vi "Connection Loop.vi"(8 "Timeout":i32=1000, 11 "connection ID":refnum<k5>) -> ()   [LabVIEW 2017]
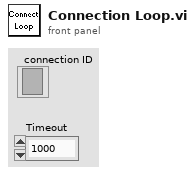
[diagram p1: front panel]
types:
  T1 = enum16{"Add Cnx", "Remove Cnx", "Retrieve List", "Cnx Inited"}
  T2 = cluster{"vi reference":refnum<vi>, "connection ID":refnum<k5>, cluster{"RPC field ID":u16, "Unique ID":u16}}
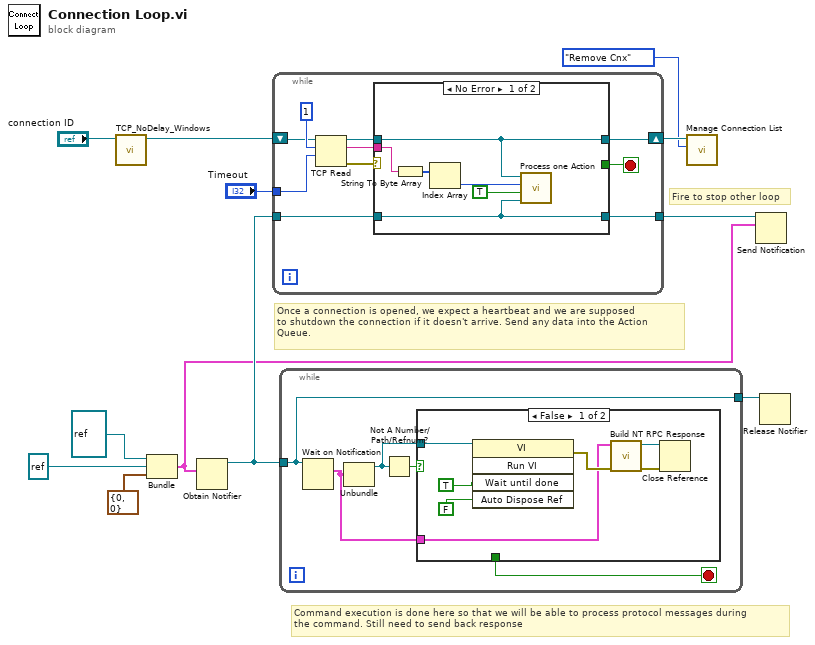
[diagram p0: block diagram]
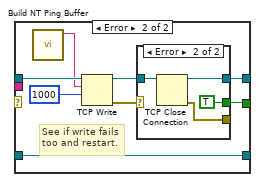
[diagram p3: hidden frame]
diagram:
  # "Command execution is done here so that we will be able to process protocol messages during\nthe command. Still need to send back response"
  # "Fire to stop other loop"
  # "Once a connection is opened, we expect a heartbeat and we are supposed\nto shutdown the connection if it doesn't arrive. Send any data into the Action\nQueue."
  n1 = call <vilib>:"TCP_NoDelay_Windows.vi"("connID"="connection ID") -> ("connID 2"=w1:refnum<k5>)  [unwired: 5 in, 1 out]
  n2 = Bundle("vi reference"=refnum<vi> refnum, "connection ID"=refnum<k5> refnum, cluster{"RPC field ID":u16, "Unique ID":u16} {"RPC field ID"=0, "Unique ID"=0}) -> (w5:T2)  [unwired: 1 in]
  n3 = Obtain Notifier(notification data type=w5) -> (notifier out=w9:refnum<notifier>)  [unwired: 3 in, 2 out]
  n4 = while {
    shift-right: [w15] -> w11
    shift-left: w1 -> [w21]
    tunnel: "Timeout" -> [w16]
    tunnel: w9 -> [w14]
    tunnel: [w13] -> w8
    stop <- w17 stop-if-true
    n5 = TCP Read(connection ID=w21, bytes to read=1 ("timeout ms (25000)"), 9:w16) -> (connection ID out=w18:refnum<k5>, data out=w19:string, error out=w20:errorcluster)  [unwired: 2 in]
    n6 = case shown="No Error" w20 {
      tunnel: w19 -> [w28 _]
      tunnel: [w26 w36] -> w15
      tunnel: w18 -> [w26 w34]
      tunnel: [_ w31] -> w17
      tunnel: w14 -> [w23 w29]
      tunnel: [w23 w29] -> w13
      frame No Error {
        n7 = String To Byte Array(string=w28) -> (unsigned byte array=w27:u8[])
        n8 = Index Array(array=w27) -> (element=w25:u8)  [unwired: 1 in]
        n9 = call <vilib>:"Process one Action.vi"("RPC notifier in"=w23, "Server"=TRUE, "First Byte"=w25, "connection ID"=w26) -> ()  [unwired: 6 in, 2 out]
      }
      frame Error {
        # "See if write fails\ntoo and restart."
        n10 = call <vilib>:"Build NT Ping Buffer.vi"() -> ("Data Buffer"=w30:string)  [unwired: 11 in]
        n11 = TCP Write(connection ID=w34, data in=w30, 9:1000 ("timeout ms (25000)")) -> (connection ID out=w33:refnum<k5>, error out=w32:errorcluster)  [unwired: 1 in, 1 out]
        n12 = case shown="Error" w32 {
          tunnel: w33 -> [w37 w41]
          tunnel: [w37 w40] -> w36
          tunnel: [_ TRUE] -> w31
          tunnel: [_ w38] -> _
          frame No Error {
          }
          frame Error {
            n13 = TCP Close Connection(connection ID=w41) -> (connection ID out=w40:refnum<k5>, error out=w38:errorcluster)  [unwired: 2 in]
          }
        }
      }
    }
  }
  n14 = while {
    tunnel: w9 -> [w44]
    tunnel: [w44] -> w7
    stop <- w45 stop-if-true
    n15 = Wait on Notification(notifier=w44) -> (notification=w42:T2)  [unwired: 3 in, 3 out]
    n16 = Unbundle(w42) -> ("vi reference"=w43:refnum<vi>)  [unwired: 2 out]
    n17 = Not A Number/Path/Refnum?(number/path/refnum=w43) -> (NaN/Path/Refnum?=w46:bool)
    n18 = case shown="False" w46 {
      selector: w46 -> [_ w54]
      tunnel: w43 -> [w51 _]
      tunnel: [_ w54] -> w45
      tunnel: w42 -> [w47 _]
      frame False {
        n19 = invoke class="VI" method="Run VI"(reference=w51, "Wait until done"=TRUE ("Wait Until Done"), "Auto Dispose Ref"=FALSE ("Wait Until Done")) -> (error out=w50:errorcluster)  [unwired: 2 in, 4 out]
        n20 = call <vilib>:"Build NT RPC Response.vi"("error in (no error)"=w50, "RPC Info"=w47) -> ("error out"=w48:errorcluster, "VI out"=w49:refnum<vi>)  [unwired: 8 in]
        n21 = Close Reference(reference=w49, error in (no error)=w48) -> ()  [unwired: 1 out]
      }
      frame True {
      }
    }
  }
  n22 = call <vilib>:"Manage Connection List.vi"("Operation"=T1."Remove Cnx", "connection ID"=w11) -> ()  [unwired: 7 in, 3 out]
  n23 = Send Notification(notification=w5, notifier=w8) -> ()  [unwired: 1 in, 2 out]
  n24 = Release Notifier(notifier=w7) -> ()  [unwired: 2 in, 3 out]
